vi "List ID.vi"(7 "Tree ID":string, 8 "Error In":errorcluster, 11 "Tree Manager":refnum<data-value>) -> (0 "Error Out":errorcluster, 1 "Child Names":string[](array[string]), 3 "Tree Manager":refnum<data-value>, 5 "Child IDs":string[](array[string]))   [LabVIEW 2017, in "Tree API.lvlib" / "Tree.lvclass"]
doc: "List the direct Children of the wired in Parent Tree. If the Parent ID input is left unwired all Trees ID are listed.\n\nThe list order is random if listing all Trees and as defined when listing Children of a specific Tree."
uses:
  Tree.lvclass
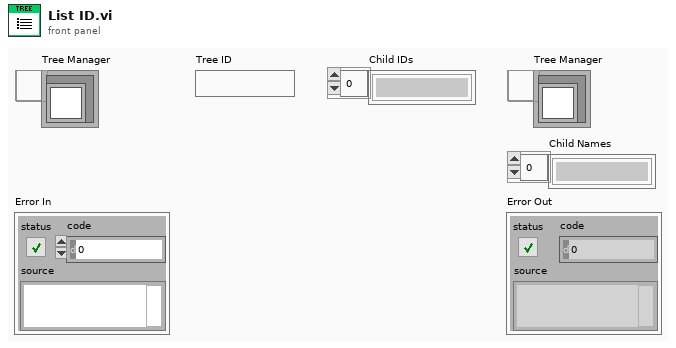
[diagram p1: front panel]
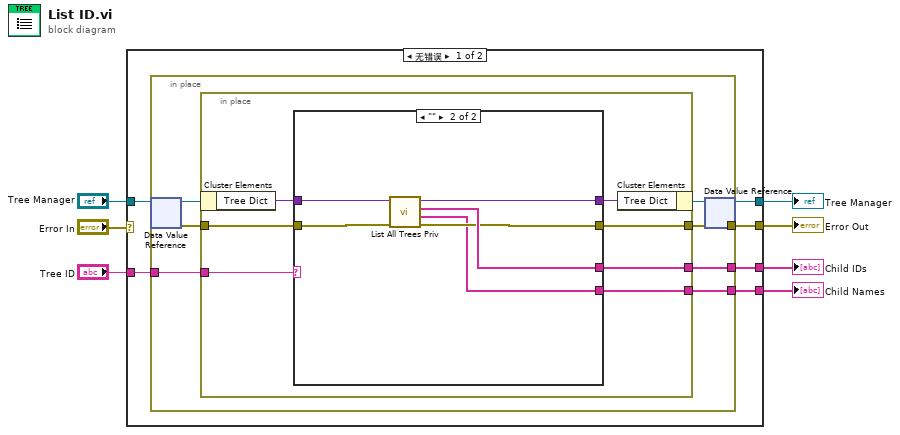
[diagram p0: block diagram]
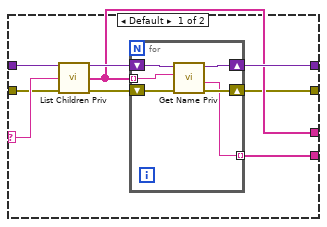
[diagram p2: hidden frame]
diagram:
  n1 = case shown="无错误" "Error In" {
    selector: "Error In" -> [_ w49]
    tunnel: "Tree Manager" -> [w13 w50]
    tunnel: [w12 w50] -> w6
    tunnel: [w8 w49] -> w4
    tunnel: "Tree ID" -> [w11 _]
    tunnel: [w10 _] -> w2
    tunnel: [w9 _] -> w1
    frame No Error {
      n2 = in-place {
        in-place-border: w11 -> [w17]
        in-place-border: [w16] -> w10
        in-place-border: [w15] -> w9
        in-place-border: [w14] -> w8
        n3 = in-place-dvr #1(w13) -> (w20:refnum<class "Tree.lvclass">, w18:errorcluster)
        n4 = in-place {
          in-place-border: w18 -> [w26]
          in-place-border: w17 -> [w25]
          in-place-border: [w23] -> w16
          in-place-border: [w22] -> w15
          in-place-border: [w21] -> w14
          n5 = in-place-cluster #2(w20) -> ("Tree Dict"=w27:variant)
          n6 = case shown="\"\"" w25 {
            selector: w25 -> [w35 _]
            tunnel: w27 -> [w36 w48]
            tunnel: w26 -> [w34 w47]
            tunnel: [w31 w45] -> w24
            tunnel: [w29 w46] -> w23
            tunnel: [w30 w43] -> w22
            tunnel: [w28 w44] -> w21
            frame Default {
              n7 = call "List Children Priv.vi"("Tree Dictionary"=w36, "Parent ID"=w35, "Error In"=w34) -> ("Tree Dictionary Out"=w33:variant, "Child IDs"=w29:string[], "Error Out"=w32:errorcluster)  [unwired: 10 in]
              n8 = for {
                shift-right: [w41] -> w31
                shift-left: w33 -> [w42]
                tunnel: w29 -> [w39] mode=indexing
                shift-right: [w38] -> w28
                shift-left: w32 -> [w40]
                tunnel: [w37] -> w30 mode=indexing
                n9 = call "Get Name Priv.vi"("error in"=w40, "Unique ID"=w39, "Tree Dictionary"=w42) -> ("error out"=w38:errorcluster, "Name"=w37:string, "Tree Dictionary Out"=w41:variant)  [unwired: 6 in]
              }
            }
            frame "" {
              n10 = call "List All Trees Priv.vi"("error in"=w47, "Tree Dict"=w48) -> ("error out"=w44:errorcluster, "Tree Names"=w43:string[], "Tree IDs"=w46:string[], "Tree Dict"=w45:variant)  [unwired: 6 in]
            }
          }
          n11 = in-place-cluster #2("Tree Dict"=w24) -> (w19:refnum<class "Tree.lvclass">)
        }
        n12 = in-place-dvr #1(w19) -> (w12:refnum<data-value>)  [unwired: 1 out]
      }
    }
    frame Error {
    }
  }
  "Tree Manager" <- w6
  "Error Out" <- w4
  "Child IDs" <- w2
  "Child Names" <- w1
